vi "Raw_BG_corrSD.vi"(2 "raw bg":i32[](array[numeric]), 3 "Data Raw":i32[][][][](array[numeric])) -> (0 "Data corrected":dbl[][](array[numeric]))   [LabVIEW 2020]
uses:
  average-2Darray-SD_int.vi
  average-2Darray-SD_double.vi
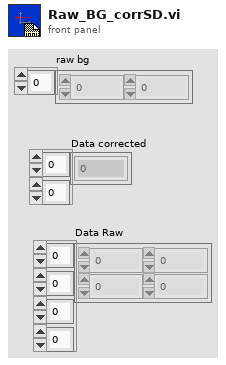
[diagram p1: front panel]
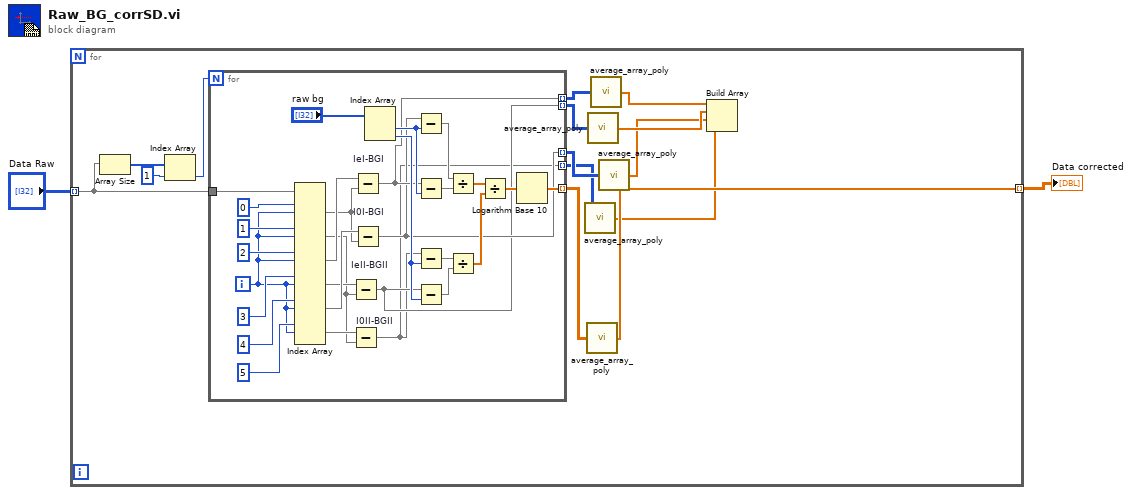
[diagram p0: block diagram]
diagram:
  n1 = for {
    tunnel: "Data Raw" -> [w13] mode=indexing
    tunnel: [w11] -> w1 mode=indexing
    n2 = Array Size(array=w13) -> (size(s)=w16:i32[])
    n3 = Index Array(array=w16, index=1) -> (element=w14:i32)
    n4 = for {
      N: w14 -> [_]
      tunnel: w13 -> [w45]
      tunnel: [w28] -> w12 mode=indexing
      tunnel: [w20] -> w10 mode=indexing
      tunnel: [w19] -> w8 mode=indexing
      tunnel: [w18] -> w9 mode=indexing
      tunnel: [w17] -> w7 mode=indexing
      i -> [w38]
      n5 = Index Array(array=w45, index (dim 0) #1=0 ("disabled index (page)"), index (dim 1) #1=w38, index (dim 0) #2=1 ("index (page)"), index (dim 1) #2=w38, index (dim 0) #3=2 ("index (page)"), index (dim 1) #3=w38, index (dim 0) #4=3 ("index (page)"), index (dim 1) #4=w38, index (dim 0) #5=4 ("index (page)"), index (dim 1) #5=w38, index (dim 0) #6=5 ("index (page)"), index (dim 1) #6=w38) -> (element #1=w35:i32[], element #2=w32:i32[], element #3=w37:i32[], element #4=w33:i32[], element #5=w36:i32[], element #6=w34:i32[])  [unwired: 6 in]
      n6 = Subtract "IeII-BGII"(x=w33, y=w32) -> (x-y=w18:i32[])
      n7 = Subtract "I0II-BGII"(x=w34, y=w32) -> (x-y=w17:i32[])
      n8 = Subtract "IeI-BGI"(x=w37, y=w35) -> (x-y=w20:i32[])
      n9 = Subtract "I0I-BGI"(x=w36, y=w35) -> (x-y=w19:i32[])
      n10 = Index Array(array="raw bg") -> (element #1=w22:i32, element #2=w21:i32)  [unwired: 2 in]
      n11 = Subtract(x=w19, y=w22) -> (x-y=w27:i32[])
      n12 = Subtract(x=w20, y=w22) -> (x-y=w26:i32[])
      n13 = Subtract(x=w17, y=w21) -> (x-y=w25:i32[])
      n14 = Subtract(x=w18, y=w21) -> (x-y=w24:i32[])
      n15 = Divide(x=w27, y=w26) -> (x/y=w31:dbl[])
      n16 = Divide(x=w25, y=w24) -> (x/y=w30:dbl[])
      n17 = Divide(x=w31, y=w30) -> (x/y=w29:dbl[])
      n18 = Logarithm Base 10(1:w29) -> (0:w28:dbl[])
    }
    n19 = call-poly "average_array_poly.vi"("2D array"=w7) -> ("out array"=w3:dbl[])
    n20 = call-poly "average_array_poly.vi"("2D array"=w12) -> ("out array"=w11:dbl[])
    n21 = call-poly "average_array_poly.vi"("2D array"=w9) -> ("out array"=w5:dbl[])
    n22 = call-poly "average_array_poly.vi"("2D array"=w10) -> ("out array"=w6:dbl[])
    n23 = call-poly "average_array_poly.vi"("2D array"=w8) -> ("out array"=w4:dbl[])
    n24 = Build Array(w6, w5, w4, w3) -> ()  [unwired: 1 out]
  }
  "Data corrected" <- w1
